vi "CS POLARIS BME DG Client.get i attribute.vi"(0 "i ref in":refnum<vi>, 5 "error in (no error)":errorcluster) -> (14 "i ref out":refnum<vi>, 16 "i attribute":T1, 19 "error out":errorcluster)   [LabVIEW 2009, in "CS POLARIS BME DG Client.lvlib"]
doc: "Gets the i attribute data of an object.\n\nLicense Agreement for this software:\n\nCopyright (C)\nGesellschaft für Schwerionenforschung, GSI\nPlanckstr. 1\n64291 Darmstadt\nGermany\n\nContact: D.Beck@gsi.de \n\nThis program is free software; you can redistribute it and/or modify it under the terms of the GNU General Public License as published by the Free Software Foundation; either version 2 of the license, or (at your option) any later version.\n\nThis program is distributed in the hope that it will be useful, but WITHOUT ANY WARRANTY; without even the implied warranty of MERCHANTABILITY or FITNESS FOR A PARTICULAR PURPOSE. See the GNU General License for more details (http://www.gnu.org).\n\nGesellschaft für Schwerionenforschung, GSI\nPlanckstr. 1, 64291 Darmstadt, Germany\nFor all questions and ideas contact: M.Richter@gsi.de, H.Brand@gsi.de or D.Beck@gsi.de.\nLast update: 17-JUN-2004"
uses:
  CS POLARIS BME DG Client.lvlib
  CS POLARIS BME DG Client.i attribute.ctl
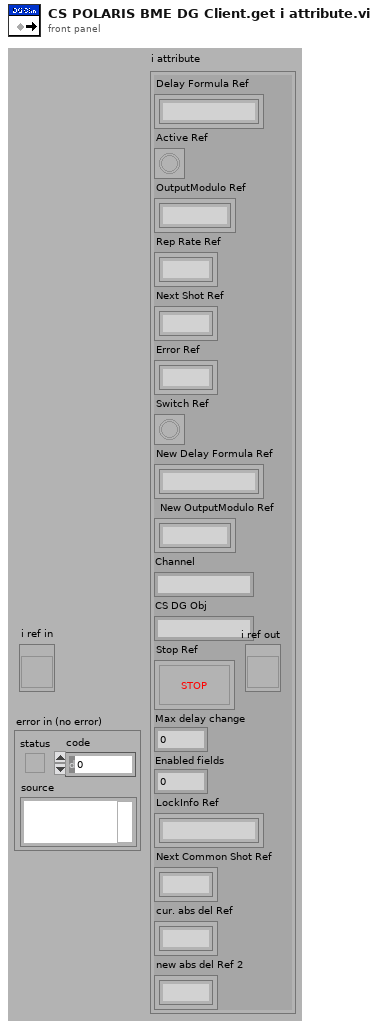
[diagram p1: front panel]
types:
  T1 = typedef "CS POLARIS BME DG Client.lvlib/CS POLARIS BME DG Client.i attribute.ctl" = cluster{"Delay Formula Ref":refnum<vi>, "Active Ref":refnum<vi>, "OutputModulo Ref":refnum<vi>, "Rep Rate Ref":refnum<vi>, "Next Shot Ref":refnum<vi>, "Error Ref":refnum<vi>, "Switch Ref":refnum<vi>, "New Delay Formula Ref":refnum<vi>, "New OutputModulo Ref ":refnum<vi>, "Channel":string, "CS DG Obj":string, "Stop Ref":refnum<vi>, "Max delay change":dbl, "Enabled fields":u8, "LockInfo Ref":refnum<vi>, "Next Common Shot Ref":refnum<vi>, "cur. abs del Ref":refnum<vi>, "new abs del Ref 2":refnum<vi>}
  T2 = enum16{"SetAttribute", "GetAttribute", "CreateAttribute", "DestroyAttribute", "DestroyAllAtributes"}
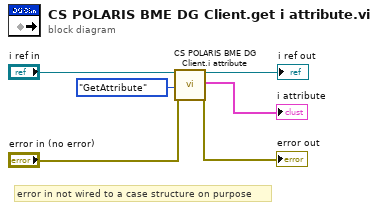
[diagram p0: block diagram]
diagram:
  # "error in not wired to a case structure on purpose"
  n1 = call "CS POLARIS BME DG Client.i attribute.vi"("VI Refnum"="i ref in", "Action"=T2."GetAttribute", "error in (no error)"="error in (no error)") -> ("VI Refnum out"=→"i ref out":refnum<vi>, "CLASS.i attribute out"=→"i attribute":T1, "error out"=→"error out":errorcluster)  [unwired: 14 in]
